vi "List Objects.vi"(7 "Max keys":u32, 8 "error in (no error)":errorcluster, 9 "Bucket":string) -> (0 "error out":errorcluster, 3 "Contents":T1[](array[typedef]))   [LabVIEW 2011, in "LV Interface for Amazon S3.lvlib"]
doc: "This operation <B>returns some or all (default)</B> of the <B>objects</B> in a bucket. To use this operation, you <B>must have READ access</B> to the bucket."
uses:
  LV Interface for Amazon S3.lvlib
  Typedefs/AMZ_S3_API_ListBucketResult Content.ctl
  Typedefs/AMZ_S3_Storage Class.ctl
  Typedefs/AMZ_S3_API_Owner.ctl
  Typedefs/AMZ_S3_API_GET Bucket Request Parameters.ctl
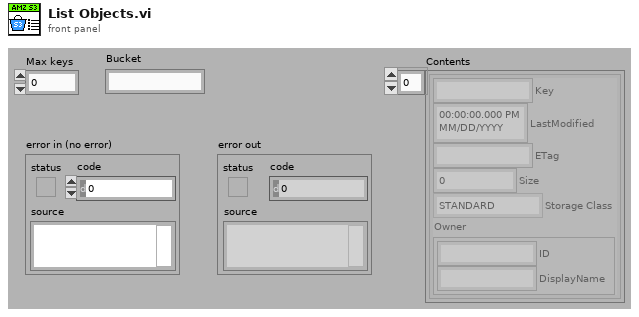
[diagram p1: front panel]
types:
  T1 = typedef "LV Interface for Amazon S3.lvlib/AMZ_S3_API_ListBucketResult Content.ctl" = cluster{"Key":string, "LastModified":timestamp, "ETag":string, "Size":u64, "Storage Class":T2, "Owner":T3}
  T2 = typedef "LV Interface for Amazon S3.lvlib/AMZ_S3_Storage Class.ctl" = enum16{"STANDARD", "REDUCED_REDUNDANCY"}
  T3 = typedef "LV Interface for Amazon S3.lvlib/AMZ_S3_API_Owner.ctl" = cluster{"ID":string, "DisplayName":string}
  T4 = typedef "LV Interface for Amazon S3.lvlib/AMZ_S3_API_GET Bucket Request Parameters.ctl" = cluster{"delimiter":string, "marker":string, "max-keys":u16, "prefix":string}
  T5 = typedef "LV Interface for Amazon S3.lvlib/AMZ_S3_API_ListBucketResult.ctl" = cluster{"Name":string, "Prefix":string, "Marker":string, "MaxKeys":u16, "IsTruncated?":bool, "Contents":T1[], "CommonPrefixes":T6[]}
  T6 = typedef "LV Interface for Amazon S3.lvlib/AMZ_S3_API_ListBucketResult CommonPrefix.ctl" = cluster{"Prefix":string}
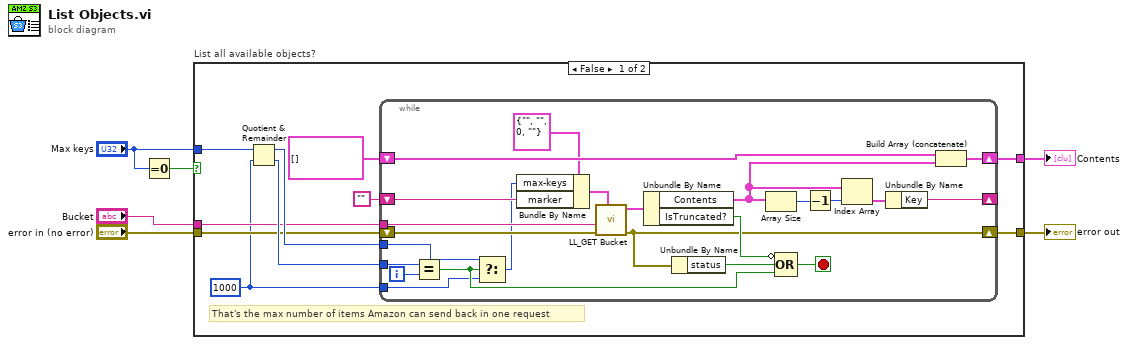
[diagram p0: block diagram]
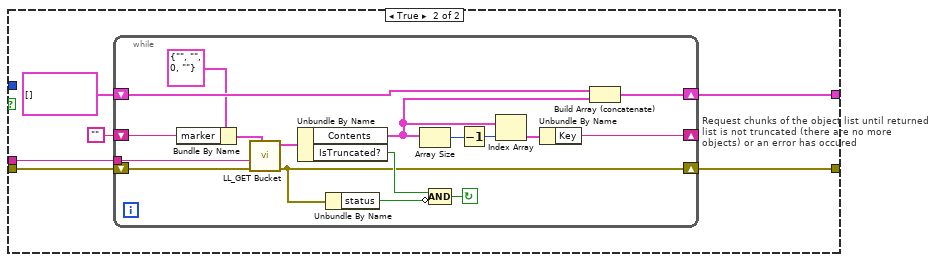
[diagram p2: hidden frame]
diagram:
  n1 = Equal To 0?(x="Max keys") -> (x = 0?=w6:bool)
  n2 = case "List all available objects?" shown="False" w6 {
    tunnel: "error in (no error)" -> [w11 w45]
    tunnel: "Max keys" -> [w16 _]
    tunnel: "Bucket" -> [w10 w44]
    tunnel: [w8 w42] -> w1
    tunnel: [w9 w40] -> w2
    frame False {
      w7 = u32 1000 ("y")
      # "That's the max number of items Amazon can send back in one request"
      n3 = Quotient & Remainder(x=w16, y=w7) -> (x-y*floor(x/y)=w12:u32, floor(x/y)=w13:u32)
      n4 = while {
        tunnel: w10 -> [w38]
        shift-right: [w34] -> w9
        shift-left: w11 -> [w39]
        shift-right: [w30] -> _
        shift-left: "" -> [w25]
        shift-right: [w28] -> w8
        shift-left: T1[] [] -> [w27]
        tunnel: w13 -> [w22]
        tunnel: w12 -> [w21]
        tunnel: w7 -> [w17]
        i -> [w23]
        stop <- w19 stop-if-true
        n5 = Equal?(x=w22, y=w23) -> (x = y?=w20:bool)
        n6 = Select(t=w21, s=w20, f=w17) -> (s? t:f=w18:u32)
        n7 = Bundle By Name(cluster=T4 {"delimiter"="", "marker"="", "max-keys"=0, "prefix"=""} ("GET Bucket Request Parameters"), "max-keys"=w18, "marker"=w25) -> (w24:T4)
        n8 = call "LL_GET Bucket.vi"("GET Bucket Request Parameters"=w24, "error in (no error)"=w39, "Bucket"=w38) -> ("error out"=w34:errorcluster, "ListBucketResult"=w37:T5)  [unwired: 6 in, 1 out]
        n9 = Unbundle By Name(w37) -> ("Contents"=w29:T1[], "IsTruncated?"=w36:bool)
        n10 = Unbundle By Name(w34) -> ("status"=w35:bool)
        n11 = Array Size(array=w29) -> (size(s)=w33:i32)
        n12 = Compound Arithmetic op=OR(invert w36, w35, w20) -> (w19:bool)
        n13 = Decrement(x=w33) -> (x-1=w32:i32)
        n14 = Index Array(array=w29, index=w32) -> (element=w31:T1)
        n15 = Unbundle By Name(w31) -> ("Key"=w30:string)
        n16 = Build Array (concatenate)(w27, w29) -> (w28:T1[])
      }
    }
    frame True {
      n17 = while "Request chunks of the object list until returned list is not truncated (there are no more objects) or an error has occured" {
        tunnel: w44 -> [w61]
        shift-right: [w56] -> w40
        shift-left: w45 -> [w62]
        shift-right: [w52] -> _
        shift-left: "" -> [w47]
        shift-right: [w50] -> w42
        shift-left: T1[] [] -> [w49]
        stop <- w57 continue-if-true
        n18 = Bundle By Name(cluster=T4 {"delimiter"="", "marker"="", "max-keys"=0, "prefix"=""} ("GET Bucket Request Parameters"), "marker"=w47) -> (w46:T4)
        n19 = call "LL_GET Bucket.vi"("GET Bucket Request Parameters"=w46, "error in (no error)"=w62, "Bucket"=w61) -> ("error out"=w56:errorcluster, "ListBucketResult"=w60:T5)  [unwired: 6 in, 1 out]
        n20 = Unbundle By Name(w60) -> ("Contents"=w51:T1[], "IsTruncated?"=w59:bool)
        n21 = Unbundle By Name(w56) -> ("status"=w58:bool)
        n22 = Array Size(array=w51) -> (size(s)=w55:i32)
        n23 = Compound Arithmetic op=AND(w59, invert w58) -> (w57:bool)
        n24 = Decrement(x=w55) -> (x-1=w54:i32)
        n25 = Index Array(array=w51, index=w54) -> (element=w53:T1)
        n26 = Unbundle By Name(w53) -> ("Key"=w52:string)
        n27 = Build Array (concatenate)(w49, w51) -> (w50:T1[])
      }
    }
  }
  "error out" <- w2
  "Contents" <- w1
